vi "_TreeItem.Property.Set.Dictionary.vi"(8 "error in (no error)":errorcluster, 9 "Dictionary":T1, 10 "Property Name":string, 11 "BaseNodeType":refnum<k24>) -> (0 "error out":errorcluster, 1 "Replaced":bool, 3 "BaseNodeType out":refnum<k24>)   [LabVIEW 2019, in "Advanced System Definition.lvlib"]
uses:
  SysDef API/Advanced System Definition.lvlib
  _Types/Property.Dictionary.ctl
  NationalInstruments.VeriStand.SystemStorage
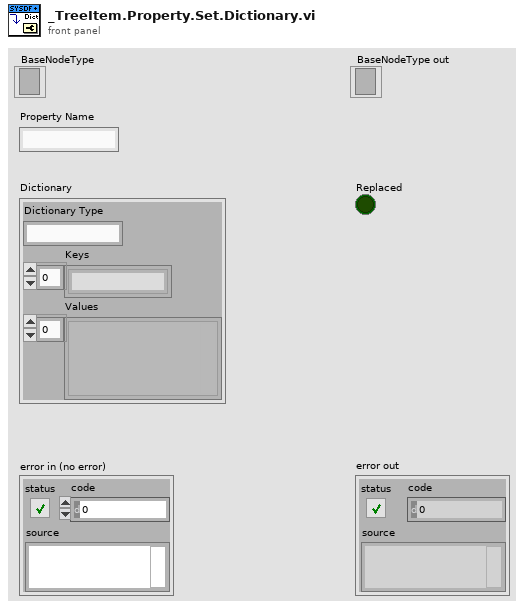
[diagram p1: front panel]
types:
  T1 = typedef "Advanced System Definition.lvlib/Property.Dictionary.ctl" = cluster{"Dictionary Type":string, "Keys":string[], "Values":variant[]}
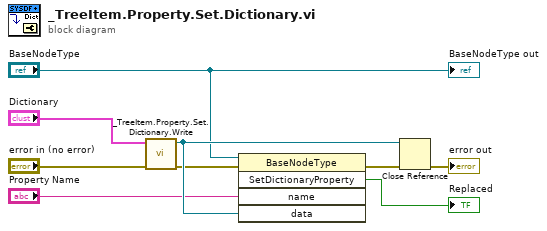
[diagram p0: block diagram]
diagram:
  n1 = call "_TreeItem.Property.Set.Dictionary.Write.vi"("error in (no error)"="error in (no error)", "Dictionary"="Dictionary") -> ("error out"=w1:errorcluster, "DictionaryProperty"=w6:refnum<k24>)  [unwired: 8 in]
  n2 = invoke class="BaseNodeType" method="SetDictionaryProperty"(reference="BaseNodeType", error in=w1, "name"="Property Name", "data"=w6) -> (error out=w7:errorcluster, "SetDictionaryProperty"=→"Replaced":bool)  [unwired: 1 in, 3 out]
  n3 = Close Reference(reference=w6, error in (no error)=w7) -> (error out=→"error out":errorcluster)
  "BaseNodeType out" <- "BaseNodeType"
